vi "transfer_station_control.vi"() -> ()   [LabVIEW 2025]
panel:
  in  "slow":bool
  in  "medium":bool
  in  "fast":bool
  in  "Home Buttons":bool=TRUE
  in  "1um":bool
  in  "Set custom increment":dbl=0.0001 min=1e-07 format="%^#_6e"
  in  "Move z to max":bool
  in  "10um":bool
  in  "set r position (degrees)":dbl min=-45.0 max=45.0 step=0.1 format="%_4f"
  in  "Emergency Stop":bool
  in  "100um":bool
  in  "set z position (m)":dbl min=0.0 max=0.012 step=0.0001 format="%#.4p"
  in  "set y position (m)":dbl min=0.0 max=0.012 step=0.0001 format="%#.4p"
  in  "set x position (m)":dbl min=0.0 max=0.012 step=0.0001 format="%.4p"
  in  "Home z":bool
  in  "Home y":bool
  in  "Home x":bool
  in  "Home r":bool
  in  "Home all axes":bool
  out "z position":dbl step=1e-06 format="%^#_4e"
  out "y position":dbl format="%^#_4e"
  out "x position":dbl format="%^#_4e"
  out "r position":dbl format="%#_4f"
  # "speed"
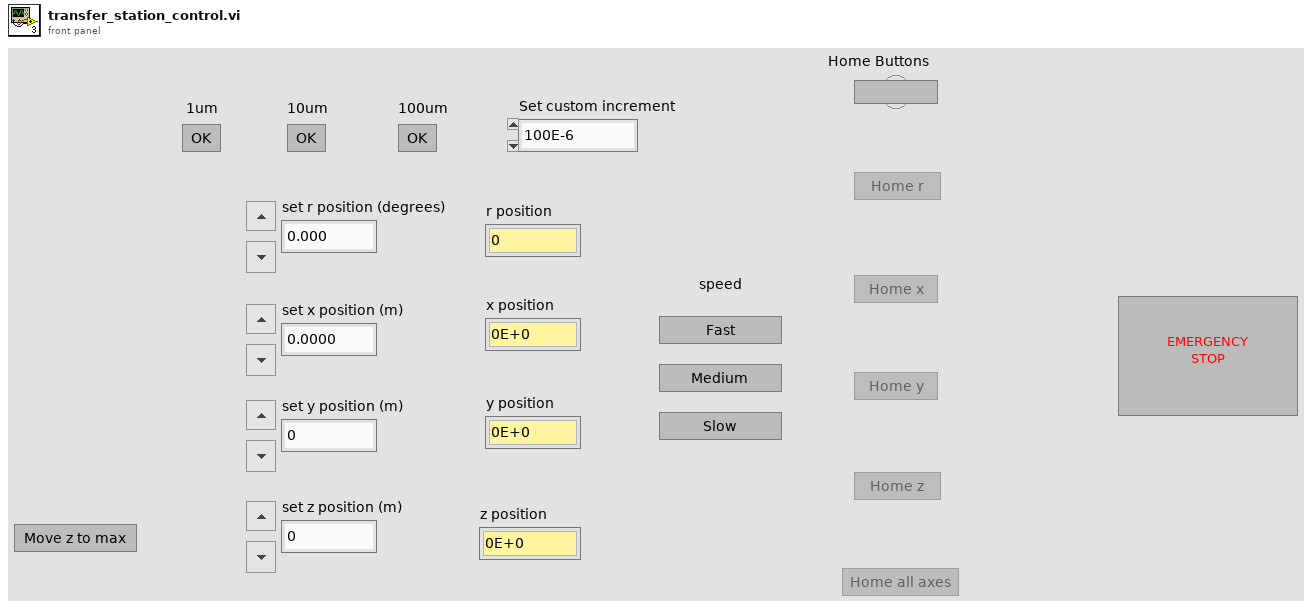
[diagram p1: front panel]
types:
  T1 = enum8{"Enabled", "Disabled", "Disabled and Grayed Out"}
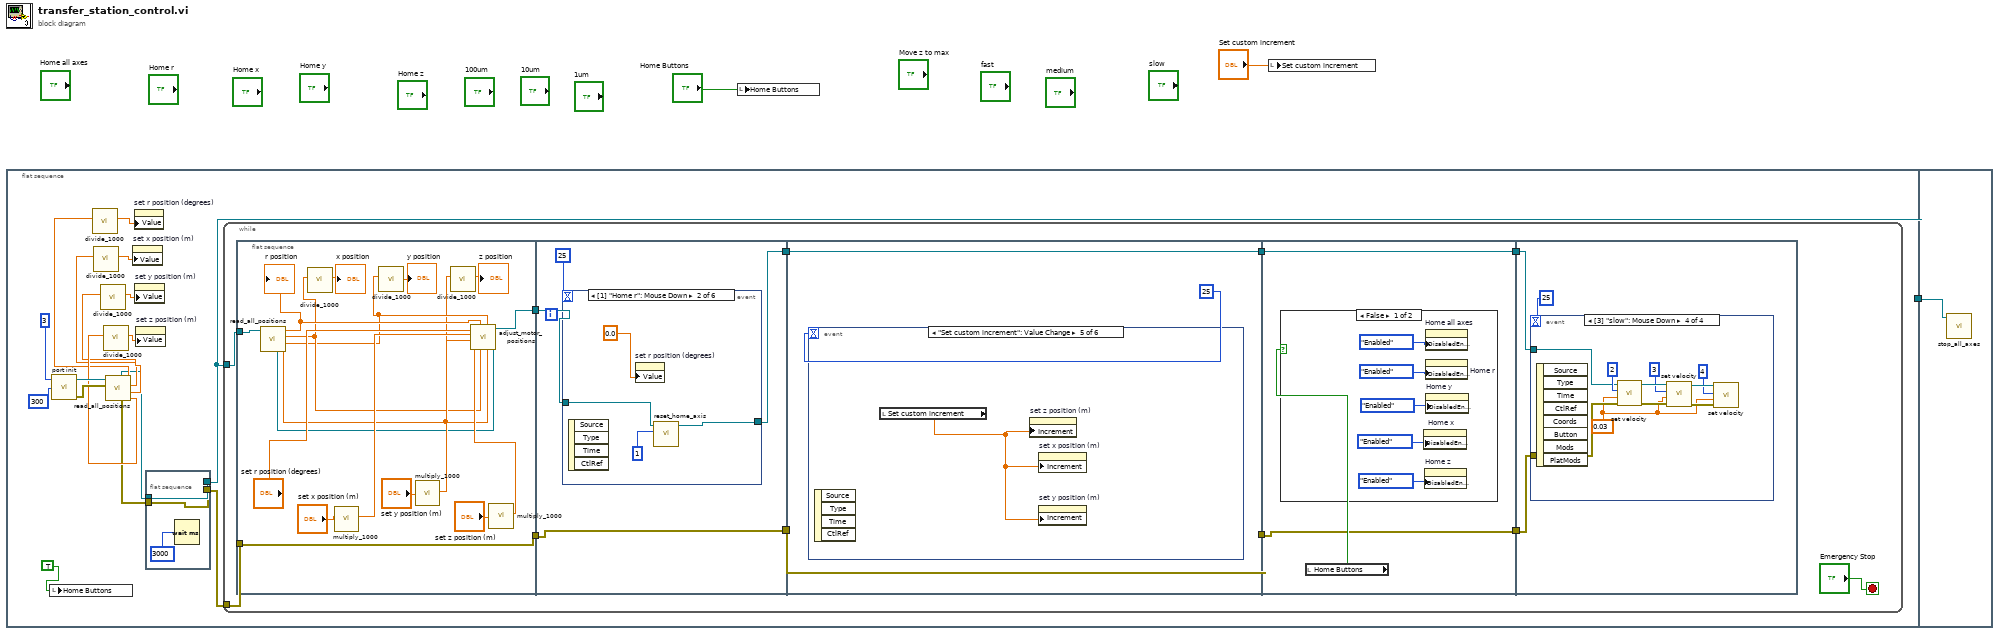
[diagram p0: block diagram]
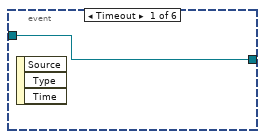
[diagram p2: hidden frame]
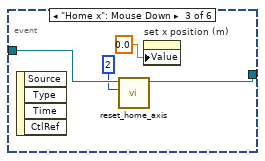
[diagram p3: hidden frame]
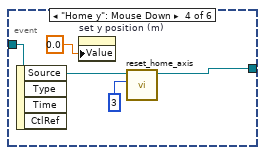
[diagram p4: hidden frame]
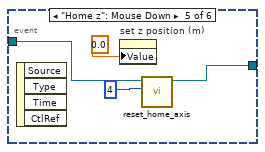
[diagram p5: hidden frame]
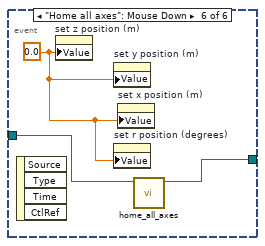
[diagram p6: hidden frame]
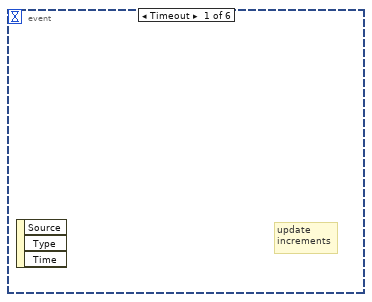
[diagram p7: hidden frame]
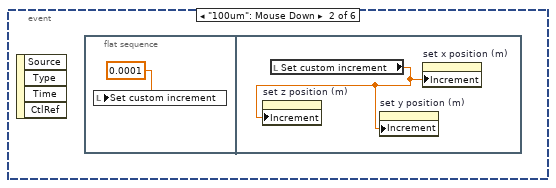
[diagram p8: hidden frame]
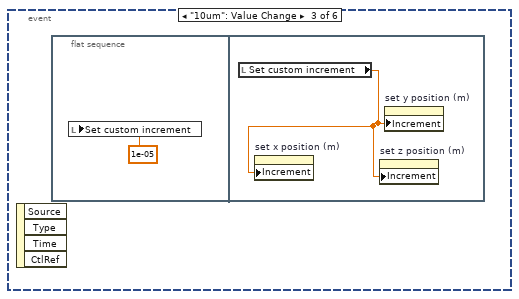
[diagram p9: hidden frame]
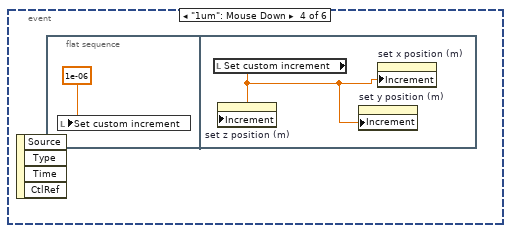
[diagram p10: hidden frame]
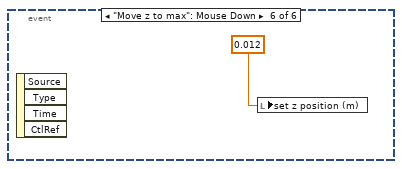
[diagram p11: hidden frame]
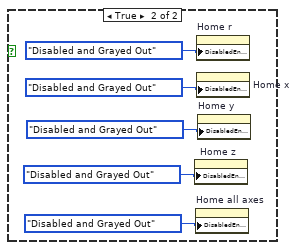
[diagram p12: hidden frame]
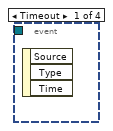
[diagram p13: hidden frame]
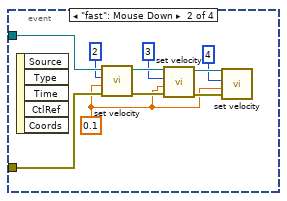
[diagram p14: hidden frame]
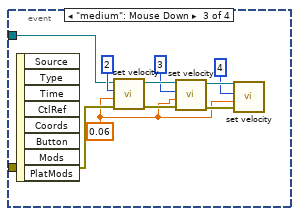
[diagram p15: hidden frame]
diagram:
  n1 = flat-sequence {
    tunnel: [w6] -> w3
    tunnel: w3 -> [w134]
    frame #0 {
      n2 = local write "Home Buttons"(TRUE ("Home Buttons")) -> ()
      n3 = call <userlib>:"port init.vi"("Timeout (ms)"=u32 300, "SerialPort"=u8 3) -> ("error out"=w17:errorcluster, "Visa Handle"=w18:refnum<visa-resource-name>)  [unwired: 2 in]
      n4 = call "read_all_positions.vi"("error in"=w17, "VISA Refnum in"=w18) -> ("z position"=w15:dbl, "y position"=w13:dbl, "x position"=w9:dbl, "r position"=w10:dbl, "error out"=w7:errorcluster, "VISA Handle out"=w8:refnum<visa-resource-name>)  [unwired: 4 in]
      n5 = call "divide_1000.vi"("Numeric"=w10) -> ("Numeric 2"=w11:dbl)  [unwired: 10 in]
      n6 = call "divide_1000.vi"("Numeric"=w9) -> ("Numeric 2"=w12:dbl)  [unwired: 10 in]
      n7 = call "divide_1000.vi"("Numeric"=w13) -> ("Numeric 2"=w14:dbl)  [unwired: 10 in]
      n8 = call "divide_1000.vi"("Numeric"=w15) -> ("Numeric 2"=w16:dbl)  [unwired: 10 in]
      n9 = property on="set x position (m)" class="DigNum (strict)"("Value"=w12) -> ()  [unwired: 2 in, 2 out]
      n10 = property on="set r position (degrees)" class="DigNum (strict)"("Value"=w11) -> ()  [unwired: 2 in, 2 out]
      n11 = property on="set y position (m)" class="DigNum (strict)"("Value"=w14) -> ()  [unwired: 2 in, 2 out]
      n12 = property on="set z position (m)" class="DigNum (strict)"("Value"=w16) -> ()  [unwired: 2 in, 2 out]
      n13 = flat-sequence {
        tunnel: w8 -> [w23]
        tunnel: [w23] -> w6
        tunnel: w7 -> [w22]
        tunnel: [w22] -> w5
        frame #0 {
          n14 = Wait (ms)(milliseconds to wait=u32 3000) -> ()  [unwired: 1 out]
        }
      }
      n15 = while {
        tunnel: w5 -> [w29]
        tunnel: w6 -> [w24]
        stop <- "Emergency Stop" stop-if-true
        n16 = flat-sequence {
          tunnel: w24 -> [w52]
          tunnel: [w51] -> w33
          tunnel: w29 -> [w35]
          tunnel: [w35] -> w28
          tunnel: w33 -> [w56]
          tunnel: [w54] -> w32
          tunnel: w28 -> [w53]
          tunnel: [w53] -> w27
          tunnel: w32 -> [w78]
          tunnel: [w78] -> w31
          tunnel: w27 -> [w77]
          tunnel: [w77] -> w26
          tunnel: w31 -> [w89]
          tunnel: [w89] -> w30
          tunnel: w26 -> [w88]
          tunnel: [w88] -> w25
          tunnel: w30 -> [w102]
          tunnel: w25 -> [w101]
          frame #0 {
            n17 = call "read_all_positions.vi"("VISA Refnum in"=w52) -> ("z position"=w38:dbl, "y position"=w40:dbl, "x position"=w42:dbl, "r position"=w50:dbl, "VISA Handle out"=w36:refnum<visa-resource-name>)  [unwired: 5 in, 1 out]
            "r position" <- w50
            n18 = call "divide_1000.vi"("Numeric"=w42) -> ("Numeric 2"=→"x position":dbl)  [unwired: 10 in]
            n19 = call "multiply_1000.vi"("Numeric"="set x position (m)") -> ("Numeric 2"=w45:dbl)  [unwired: 10 in]
            n20 = call "divide_1000.vi"("Numeric"=w40) -> ("Numeric 2"=→"y position":dbl)  [unwired: 10 in]
            n21 = call "multiply_1000.vi"("Numeric"="set y position (m)") -> ("Numeric 2"=w46:dbl)  [unwired: 10 in]
            n22 = call "divide_1000.vi"("Numeric"=w38) -> ("Numeric 2"=→"z position":dbl)  [unwired: 10 in]
            n23 = call "multiply_1000.vi"("Numeric"="set z position (m)") -> ("Numeric 2"=w48:dbl)  [unwired: 10 in]
            n24 = call "adjust_motor_positions.vi"("VISA Refnum in"=w36, "z position"=w38, "y position"=w40, "x position"=w42, "r position"=w50, "set z position"=w48, "set y position"=w46, "set x position"=w45, "set r position"="set r position (degrees)") -> ("VISA Handle out"=w51:refnum<visa-resource-name>)  [unwired: 2 in]
          }
          frame #1 {
            n25 = event shown="[1] \"Home r\": Mouse Down" {
              selector: _ -> [_ _ _ _ _ _]
              dyn-events: _ -> [_ _ _ _ _ _]
              timeout: 25 -> [_ _ _ _ _ _]
              tunnel: w56 -> [w57 w61 w65 w69 w73 w76]
              tunnel: [w57 w59 w64 w68 w72 w75] -> w54
              event Timeout {
                n26 = event-data() -> ()  [unwired: 1 in, 3 out]
              }
              event "Home r": Mouse Down {
                n27 = event-data() -> ()  [unwired: 1 in, 4 out]
                n28 = property on="set r position (degrees)" class="DigNum (strict)"("Value"=0.0 ("set r position (degrees)")) -> ()  [unwired: 2 in, 2 out]
                n29 = call "reset_home_axis.vi"("Axis in in"=1, "VISA Refnum in"=w61) -> ("VISA Handle out"=w59:refnum<visa-resource-name>)  [unwired: 6 in, 3 out]
              }
              event "Home x": Mouse Down {
                n30 = event-data() -> ()  [unwired: 1 in, 4 out]
                n31 = call "reset_home_axis.vi"("Axis in in"=2, "VISA Refnum in"=w65) -> ("VISA Handle out"=w64:refnum<visa-resource-name>)  [unwired: 6 in, 3 out]
                n32 = property on="set x position (m)" class="DigNum (strict)"("Value"=0.0 ("set x position (m)")) -> ()  [unwired: 2 in, 2 out]
              }
              event "Home y": Mouse Down {
                n33 = event-data() -> ()  [unwired: 1 in, 4 out]
                n34 = property on="set y position (m)" class="DigNum (strict)"("Value"=0.0 ("set y position (m)")) -> ()  [unwired: 2 in, 2 out]
                n35 = call "reset_home_axis.vi"("Axis in in"=3, "VISA Refnum in"=w69) -> ("VISA Handle out"=w68:refnum<visa-resource-name>)  [unwired: 6 in, 3 out]
              }
              event "Home z": Mouse Down {
                n36 = event-data() -> ()  [unwired: 1 in, 4 out]
                n37 = property on="set z position (m)" class="DigNum (strict)"("Value"=0.0 ("set z position (m)")) -> ()  [unwired: 2 in, 2 out]
                n38 = call "reset_home_axis.vi"("Axis in in"=4, "VISA Refnum in"=w73) -> ("VISA Handle out"=w72:refnum<visa-resource-name>)  [unwired: 6 in, 3 out]
              }
              event "Home all axes": Mouse Down {
                w74 = 0.0 ("set z position (m)")
                n39 = event-data() -> ()  [unwired: 1 in, 4 out]
                n40 = property on="set z position (m)" class="DigNum (strict)"("Value"=w74) -> ()  [unwired: 2 in, 2 out]
                n41 = property on="set y position (m)" class="DigNum (strict)"("Value"=w74) -> ()  [unwired: 2 in, 2 out]
                n42 = property on="set r position (degrees)" class="DigNum (strict)"("Value"=w74) -> ()  [unwired: 2 in, 2 out]
                n43 = property on="set x position (m)" class="DigNum (strict)"("Value"=w74) -> ()  [unwired: 2 in, 2 out]
                n44 = call "home_all_axes.vi"("VISA Handle in"=w76) -> ("VISA Handle out"=w75:refnum<visa-resource-name>)  [unwired: 5 in, 5 out]
              }
            }
          }
          frame #2 {
            n45 = event shown="[4] \"Set custom increment\": Value Change" {
              selector: _ -> [_ _ _ _ _ _]
              dyn-events: _ -> [_ _ _ _ _ _]
              timeout: 25 -> [_ _ _ _ _ _]
              event Timeout {
                # "update\nincrements"
                n46 = event-data() -> ()  [unwired: 1 in, 3 out]
              }
              event "100um": Mouse Down {
                n47 = event-data() -> ()  [unwired: 1 in, 4 out]
                n48 = flat-sequence {
                  frame #0 {
                    n49 = local write "Set custom increment"(0.0001 ("Data Entry Limits:Increment")) -> ()
                  }
                  frame #1 {
                    n50 = local read "Set custom increment"() -> (w81:dbl)
                    n51 = property on="set z position (m)" class="DigNum (strict)"("Increment"=w81) -> ()  [unwired: 2 in, 2 out]
                    n52 = property on="set y position (m)" class="DigNum (strict)"("Increment"=w81) -> ()  [unwired: 2 in, 2 out]
                    n53 = property on="set x position (m)" class="DigNum (strict)"("Increment"=w81) -> ()  [unwired: 2 in, 2 out]
                  }
                }
              }
              event "10um": Value Change {
                n54 = event-data() -> ()  [unwired: 1 in, 4 out]
                n55 = flat-sequence {
                  frame #0 {
                    n56 = local write "Set custom increment"(1e-05 ("Data Entry Limits:Increment")) -> ()
                  }
                  frame #1 {
                    n57 = local read "Set custom increment"() -> (w83:dbl)
                    n58 = property on="set x position (m)" class="DigNum (strict)"("Increment"=w83) -> ()  [unwired: 2 in, 2 out]
                    n59 = property on="set z position (m)" class="DigNum (strict)"("Increment"=w83) -> ()  [unwired: 2 in, 2 out]
                    n60 = property on="set y position (m)" class="DigNum (strict)"("Increment"=w83) -> ()  [unwired: 2 in, 2 out]
                  }
                }
              }
              event "1um": Mouse Down {
                n61 = event-data() -> ()  [unwired: 1 in, 4 out]
                n62 = flat-sequence {
                  frame #0 {
                    n63 = local write "Set custom increment"(1e-06 ("Data Entry Limits:Increment")) -> ()
                  }
                  frame #1 {
                    n64 = local read "Set custom increment"() -> (w85:dbl)
                    n65 = property on="set z position (m)" class="DigNum (strict)"("Increment"=w85) -> ()  [unwired: 2 in, 2 out]
                    n66 = property on="set y position (m)" class="DigNum (strict)"("Increment"=w85) -> ()  [unwired: 2 in, 2 out]
                    n67 = property on="set x position (m)" class="DigNum (strict)"("Increment"=w85) -> ()  [unwired: 2 in, 2 out]
                  }
                }
              }
              event "Set custom increment": Value Change {
                n68 = event-data() -> ()  [unwired: 1 in, 4 out]
                n69 = local read "Set custom increment"() -> (w86:dbl)
                n70 = property on="set z position (m)" class="DigNum (strict)"("Increment"=w86) -> ()  [unwired: 2 in, 2 out]
                n71 = property on="set x position (m)" class="DigNum (strict)"("Increment"=w86) -> ()  [unwired: 2 in, 2 out]
                n72 = property on="set y position (m)" class="DigNum (strict)"("Increment"=w86) -> ()  [unwired: 2 in, 2 out]
              }
              event "Move z to max": Mouse Down {
                n73 = event-data() -> ()  [unwired: 1 in, 4 out]
                n74 = local write "set z position (m)"(0.012 ("set z position")) -> ()
              }
            }
          }
          frame #3 {
            n75 = local read "Home Buttons"() -> (w90:bool)
            n76 = case shown="False" w90 {
              frame False {
                n77 = property on="Home x" class="Bool (strict)"("DisabledEnum"=T1."Enabled" ("Disabled")) -> ()  [unwired: 2 in, 2 out]
                n78 = property on="Home z" class="Bool (strict)"("DisabledEnum"=T1."Enabled" ("Disabled")) -> ()  [unwired: 2 in, 2 out]
                n79 = property on="Home all axes" class="Bool (strict)"("DisabledEnum"=T1."Enabled" ("Disabled")) -> ()  [unwired: 2 in, 2 out]
                n80 = property on="Home r" class="Bool (strict)"("DisabledEnum"=T1."Enabled" ("Disabled")) -> ()  [unwired: 2 in, 2 out]
                n81 = property on="Home y" class="Bool (strict)"("DisabledEnum"=T1."Enabled" ("Disabled")) -> ()  [unwired: 2 in, 2 out]
              }
              frame True {
                n82 = property on="Home z" class="Bool (strict)"("DisabledEnum"=T1."Disabled and Grayed Out" ("Disabled")) -> ()  [unwired: 2 in, 2 out]
                n83 = property on="Home all axes" class="Bool (strict)"("DisabledEnum"=T1."Disabled and Grayed Out" ("Disabled")) -> ()  [unwired: 2 in, 2 out]
                n84 = property on="Home r" class="Bool (strict)"("DisabledEnum"=T1."Disabled and Grayed Out" ("Disabled")) -> ()  [unwired: 2 in, 2 out]
                n85 = property on="Home x" class="Bool (strict)"("DisabledEnum"=T1."Disabled and Grayed Out" ("Disabled")) -> ()  [unwired: 2 in, 2 out]
                n86 = property on="Home y" class="Bool (strict)"("DisabledEnum"=T1."Disabled and Grayed Out" ("Disabled")) -> ()  [unwired: 2 in, 2 out]
              }
            }
          }
          frame #4 {
            n87 = event shown="[3] \"slow\": Mouse Down" {
              selector: _ -> [_ _ _ _]
              dyn-events: _ -> [_ _ _ _]
              timeout: 25 -> [_ _ _ _]
              tunnel: w102 -> [_ w113 w116 w126]
              tunnel: w101 -> [_ w111 w115 w125]
              event Timeout {
                n88 = event-data() -> ()  [unwired: 1 in, 3 out]
              }
              event "fast": Mouse Down {
                w104 = 0.1 ("Velocity value (units/s)")
                n89 = event-data() -> ()  [unwired: 1 in, 5 out]
                n90 = call "set velocity.vi"("error in"=w111, "Velocity value (units/s)"=w104, "Axis in"=2, "VISA Handle in"=w113) -> ("error out"=w107:errorcluster, "VISA Handle out"=w110:refnum<visa-resource-name>)  [unwired: 2 in, 2 out]
                n91 = call "set velocity.vi"("error in"=w107, "Velocity value (units/s)"=w104, "Axis in"=3, "VISA Handle in"=w110) -> ("error out"=w108:errorcluster, "VISA Handle out"=w109:refnum<visa-resource-name>)  [unwired: 2 in, 2 out]
                n92 = call "set velocity.vi"("error in"=w108, "Velocity value (units/s)"=w104, "Axis in"=4, "VISA Handle in"=w109) -> ()  [unwired: 2 in, 4 out]
              }
              event "medium": Mouse Down {
                w114 = 0.06 ("Velocity value (units/s)")
                n93 = event-data() -> ()  [unwired: 1 in, 8 out]
                n94 = call "set velocity.vi"("error in"=w115, "Velocity value (units/s)"=w114, "Axis in"=2, "VISA Handle in"=w116) -> ("error out"=w119:errorcluster, "VISA Handle out"=w122:refnum<visa-resource-name>)  [unwired: 2 in, 2 out]
                n95 = call "set velocity.vi"("error in"=w119, "Velocity value (units/s)"=w114, "Axis in"=3, "VISA Handle in"=w122) -> ("error out"=w120:errorcluster, "VISA Handle out"=w121:refnum<visa-resource-name>)  [unwired: 2 in, 2 out]
                n96 = call "set velocity.vi"("error in"=w120, "Velocity value (units/s)"=w114, "Axis in"=4, "VISA Handle in"=w121) -> ()  [unwired: 2 in, 4 out]
              }
              event "slow": Mouse Down {
                w124 = 0.03 ("Velocity value (units/s)")
                n97 = event-data() -> ()  [unwired: 1 in, 8 out]
                n98 = call "set velocity.vi"("error in"=w125, "Velocity value (units/s)"=w124, "Axis in"=2, "VISA Handle in"=w126) -> ("error out"=w129:errorcluster, "VISA Handle out"=w132:refnum<visa-resource-name>)  [unwired: 2 in, 2 out]
                n99 = call "set velocity.vi"("error in"=w129, "Velocity value (units/s)"=w124, "Axis in"=3, "VISA Handle in"=w132) -> ("error out"=w130:errorcluster, "VISA Handle out"=w131:refnum<visa-resource-name>)  [unwired: 2 in, 2 out]
                n100 = call "set velocity.vi"("error in"=w130, "Velocity value (units/s)"=w124, "Axis in"=4, "VISA Handle in"=w131) -> ()  [unwired: 2 in, 4 out]
              }
            }
          }
        }
      }
    }
    frame #1 {
      n101 = call "stop_all_axes.vi"("VISA Refnum in"=w134) -> ()  [unwired: 11 in]
    }
  }
  n102 = local write "Home Buttons"("Home Buttons") -> ()
  n103 = local write "Set custom increment"("Set custom increment") -> ()
